vi "xml generate for SFP+_VNA_Full.vi"(0 "width1":dbl, 1 "width2":dbl, 2 "single spec":T1={"limit Spec"=array1616x8[12928 elements], "Diff Test Item Name"=["SDD21", "SDD11", "SCD22", "SCC11", "SCD21-SDD21", "NEXT", "ILD_15"], "Spec _Col"=[1, 2, 3, 4, 5, 6, 7]}, 3 "auto get refer point":bool, 4 "input_array_TDD11":string[](array[string]), 5 "input_array_TDD22":string[](array[string]), 6 "input_path_dataSource":path, 7 "input_test_results":bool[](array[boolean]), 8 "show_impspec":string[](array[string]), 10 "路径":path=path "D:/wmgxml.xml", 11 "input_array_time":string[](array[string]), 12 "input_str_label":string, 13 "input_array_impSpec":string[](array[string]), 14 "input_str_CustomerPN":string, 16 "FilePath":string, 17 "FileVer":string, 18 "terminal points":dbl[](array[numeric]), 19 "cable points":dbl[](array[numeric])) -> ()   [LabVIEW 2011]
uses:
  <vilib>/Utility/file.llb/Read From Spreadsheet File (DBL).vi
panel:
  out "terminal points 2":dbl[](array[numeric])
  out "TestResult":string
  out "TDD":string
  out "NEXT":string
  out "SCC11":string
  out "SCD21-SDD21":string
  out "ILD":string
  out "SDD11":string
  out "SDD21":string
  out "midVar_time":string[](array[string])
  in  "midVar_state":string
  in  "input_str_product":string
  out "midVar_Content":string
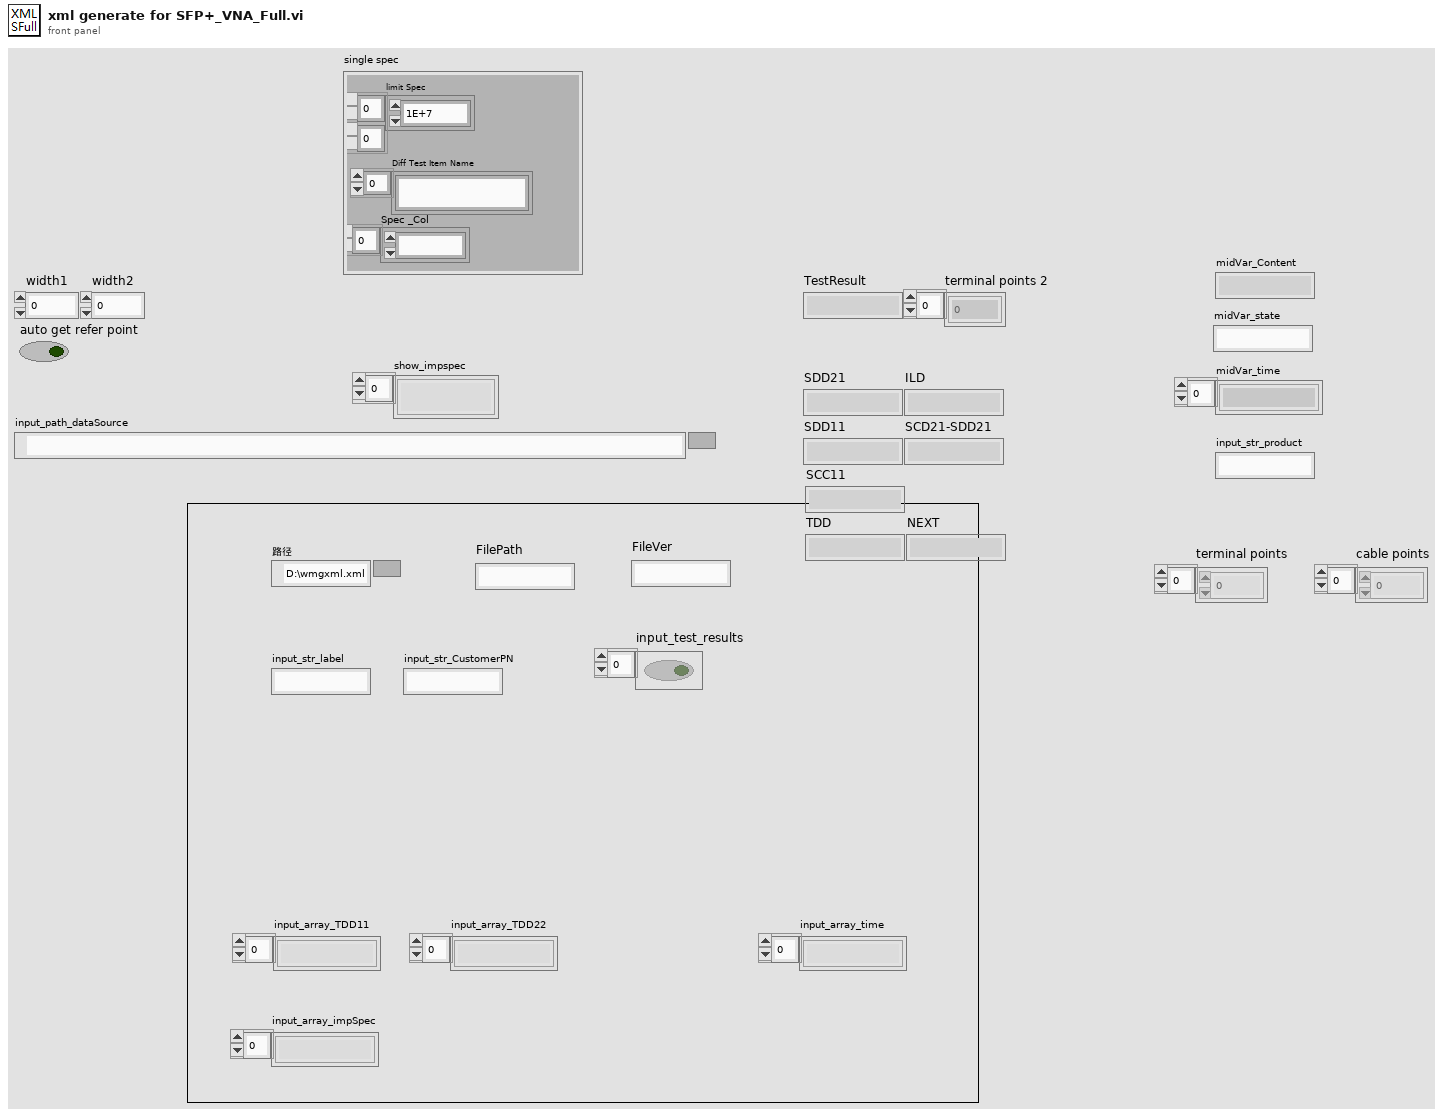
[diagram p1: front panel]
types:
  T1 = cluster{"limit Spec":dbl[][], "Diff Test Item Name":string[], "Spec _Col":i32[]}
  T2 = enum16{"open", "replace", "create", "open or create", "replace or create", "replace or create with confirmation"}
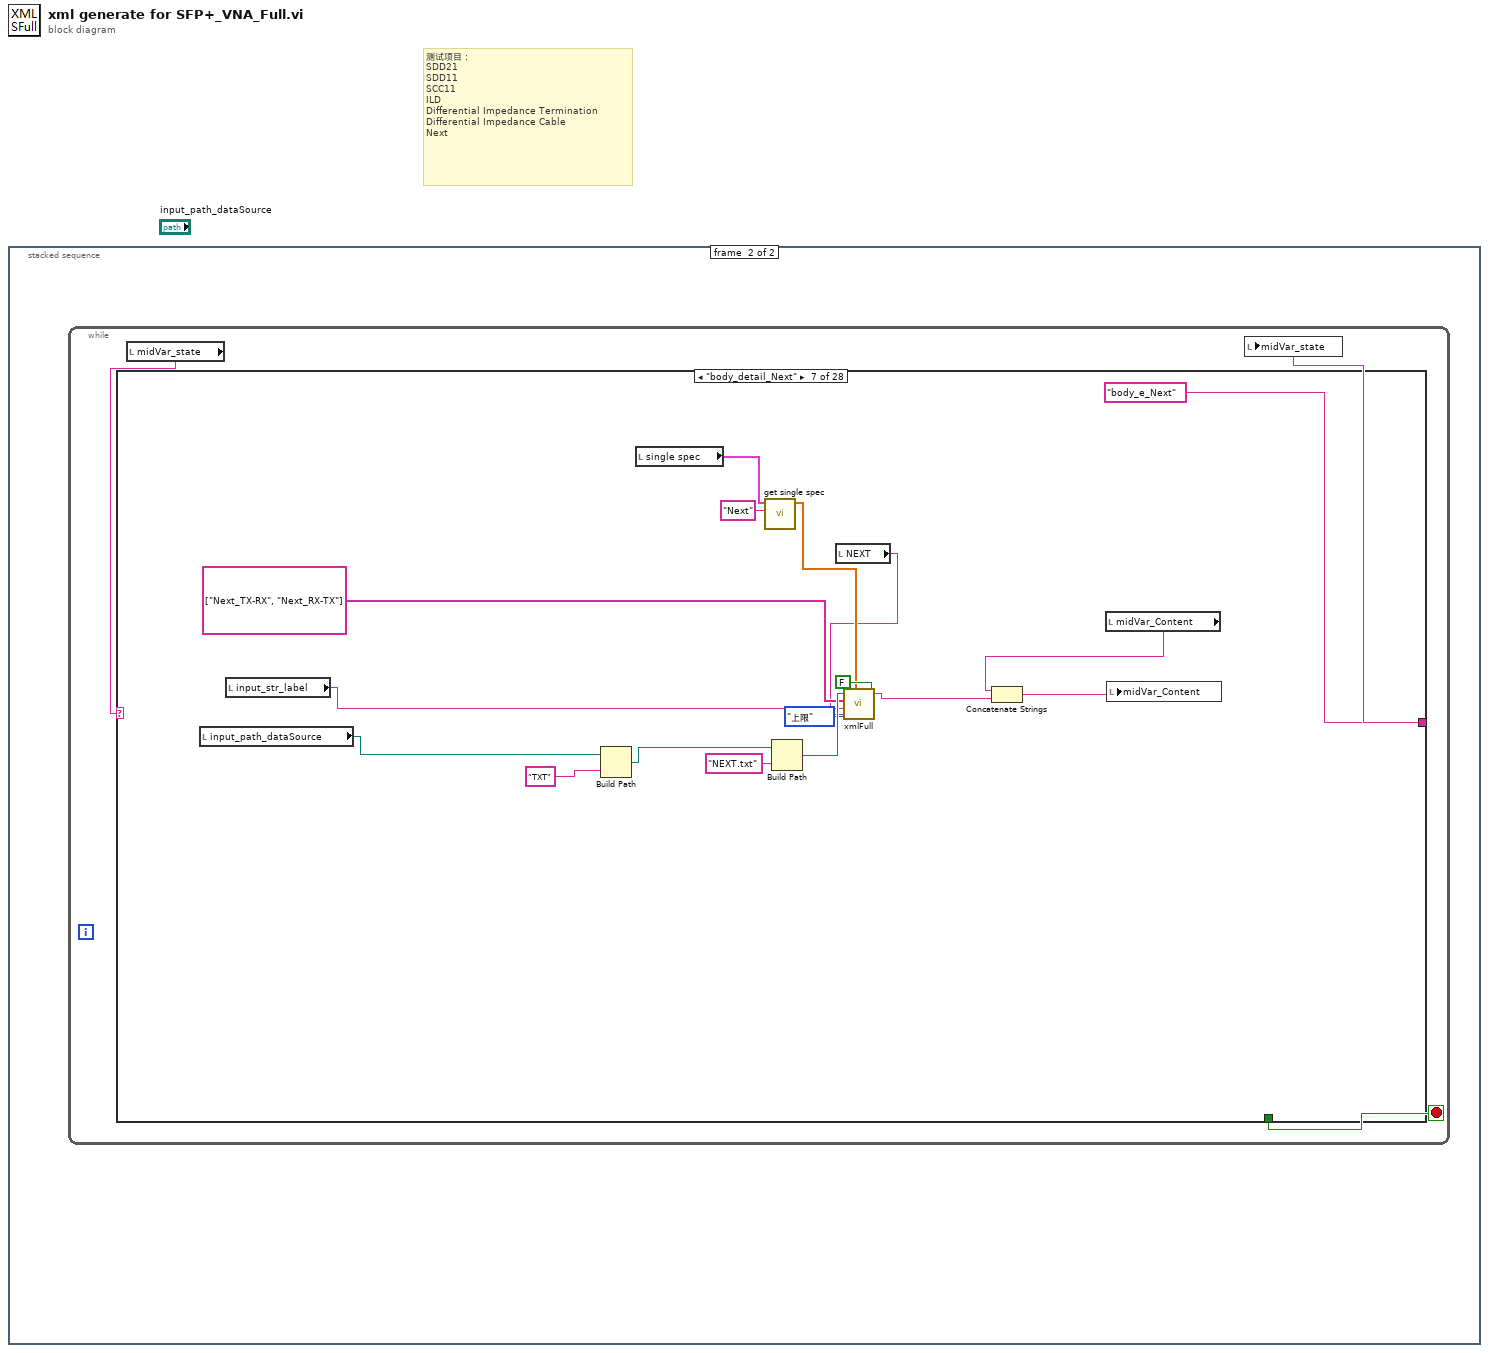
[diagram p0: block diagram]
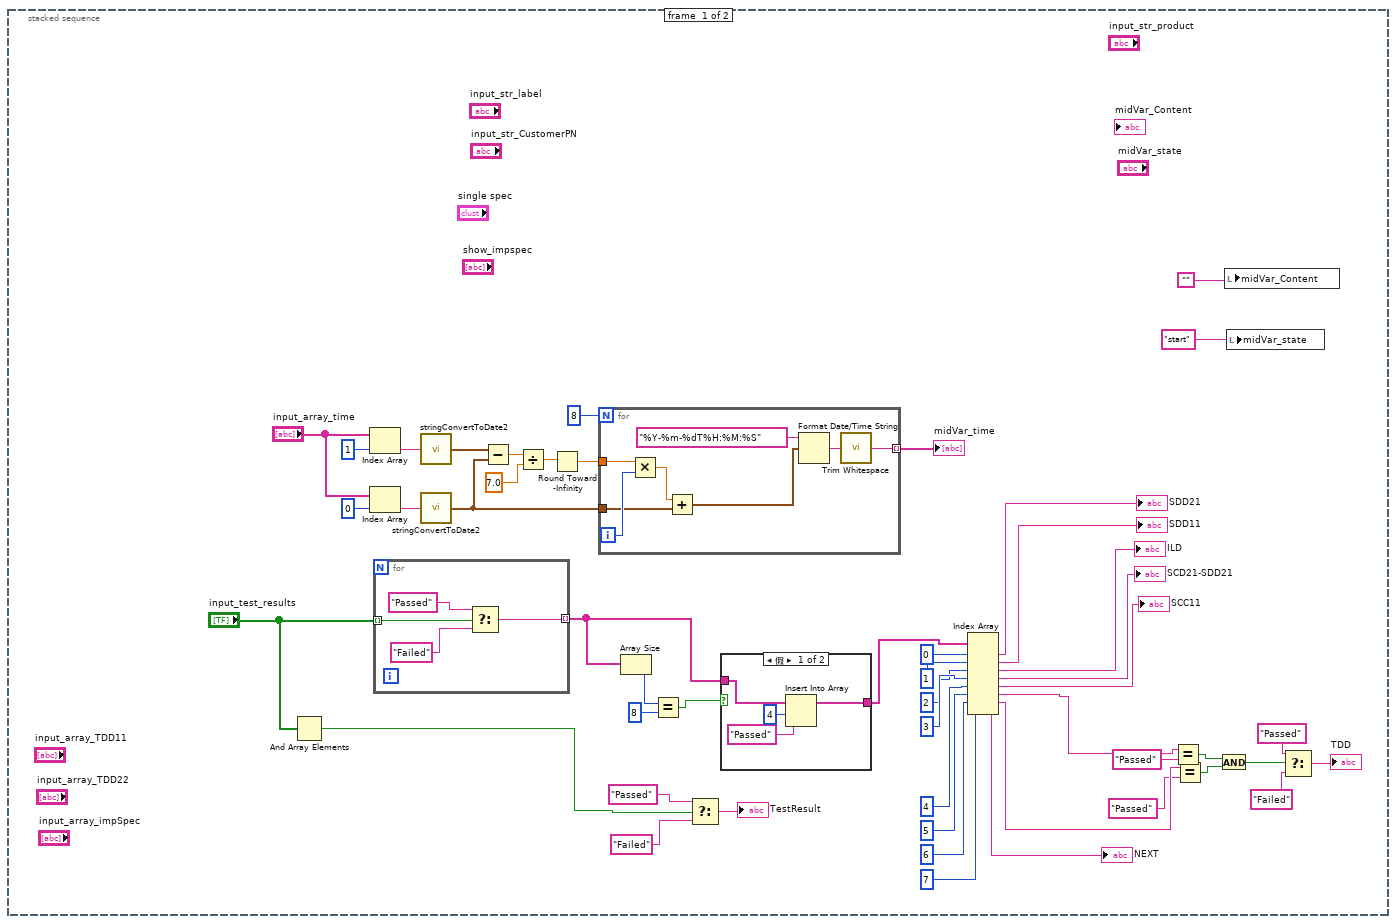
[diagram p2: hidden frame]
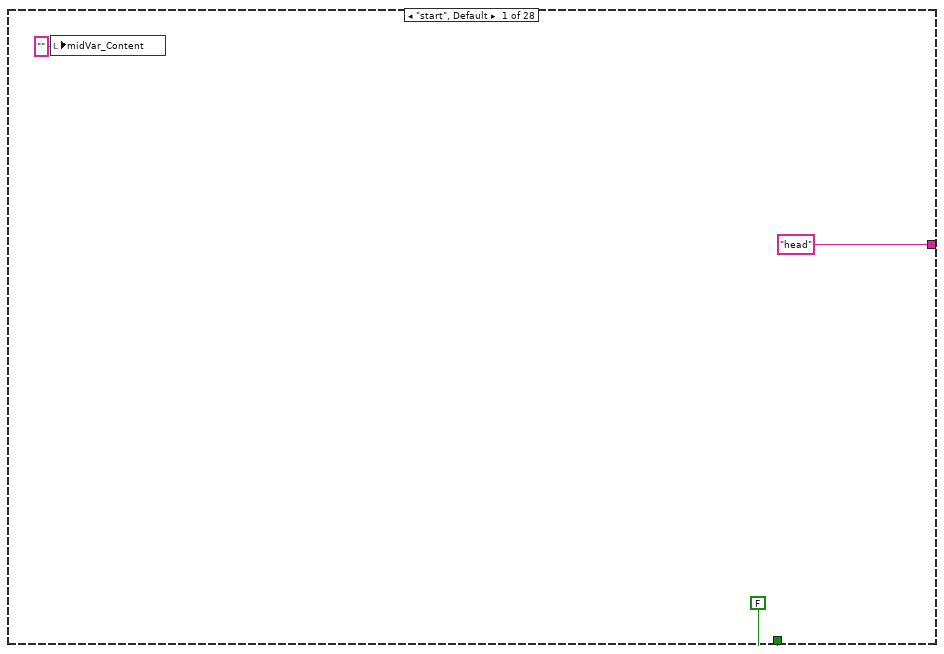
[diagram p4: hidden frame]
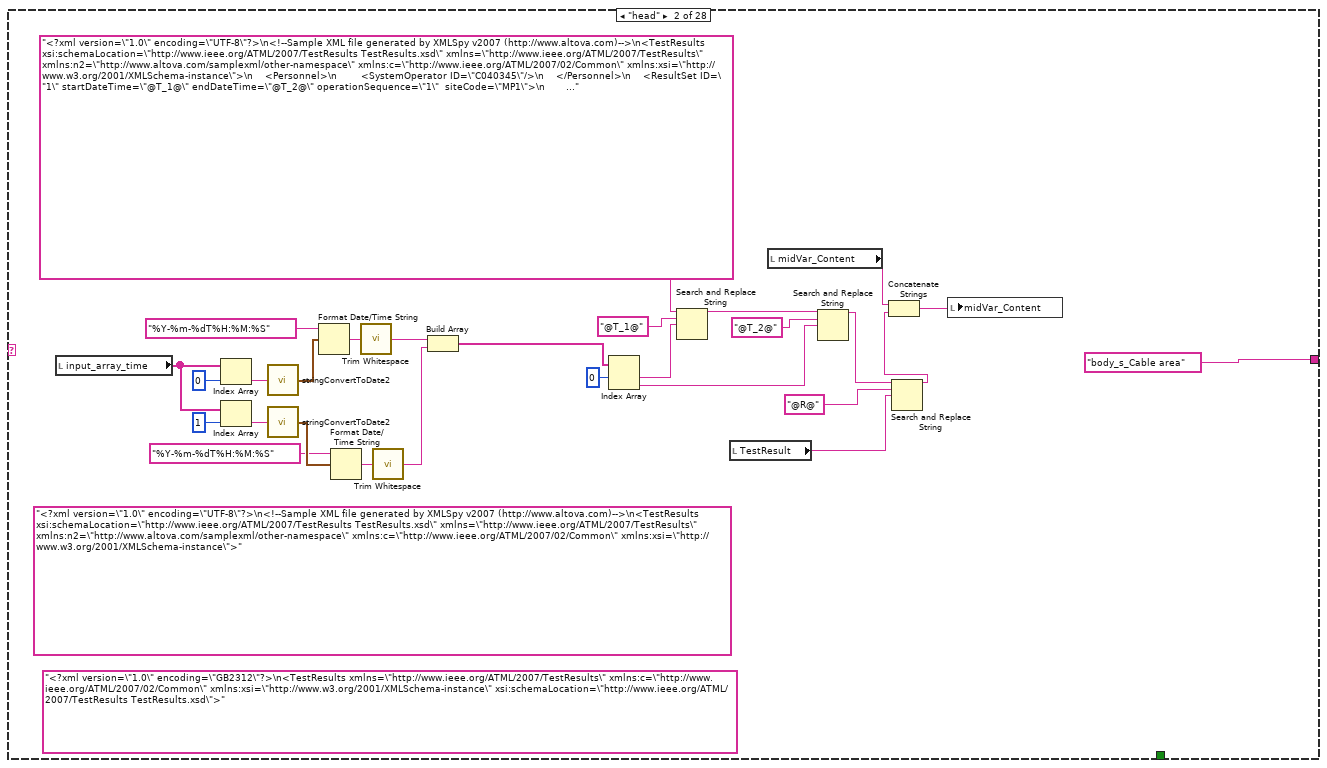
[diagram p5: hidden frame]
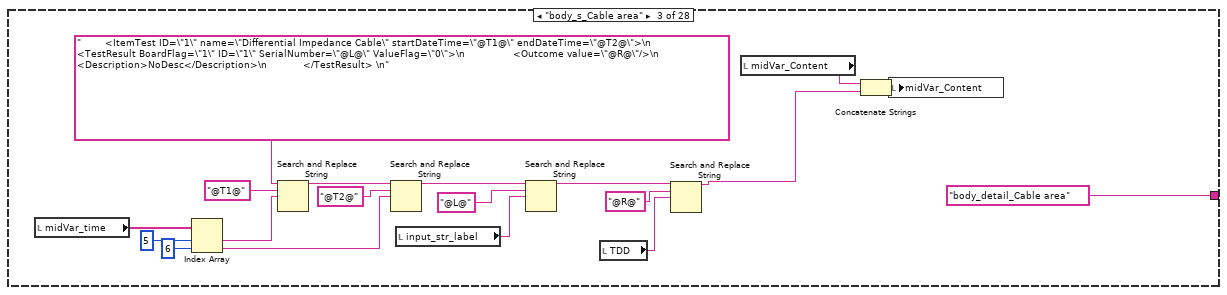
[diagram p6: hidden frame]
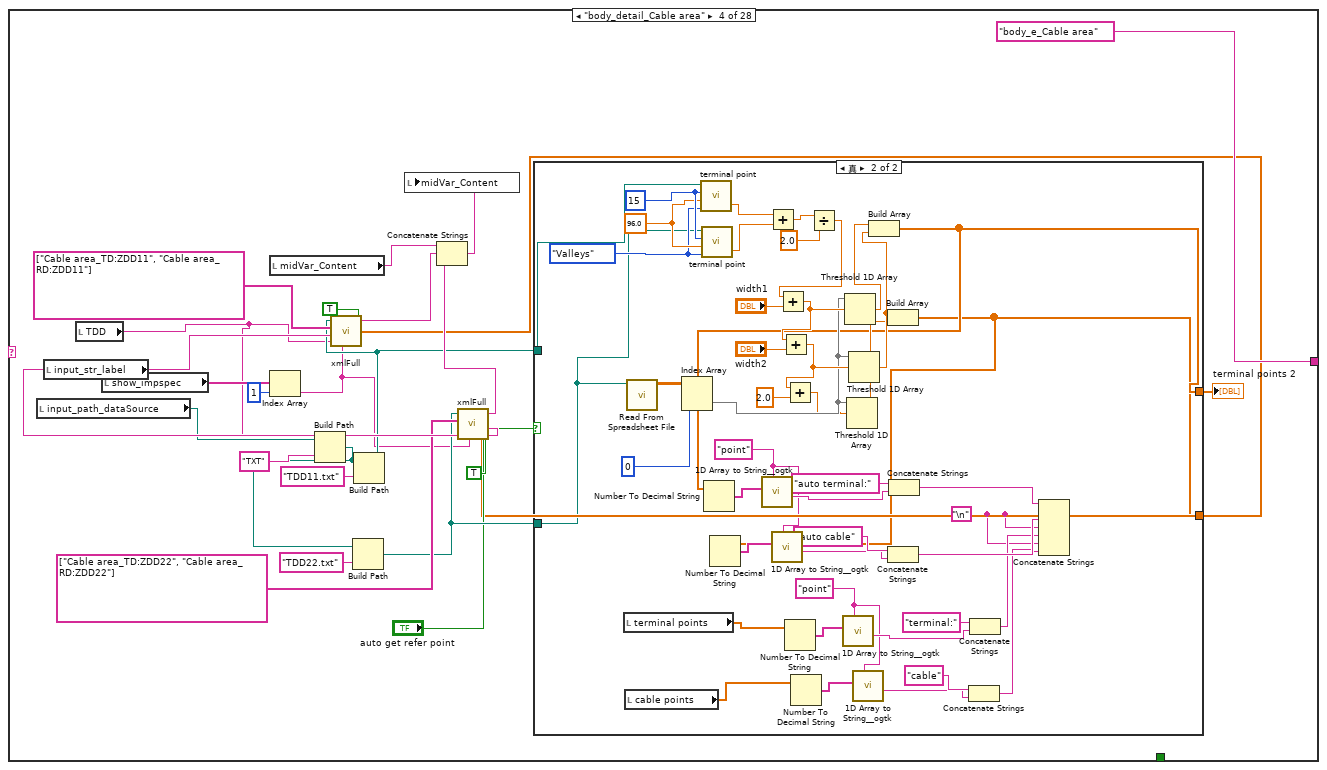
[diagram p7: hidden frame]
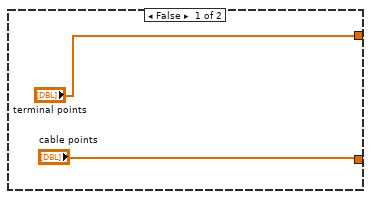
[diagram p8: hidden frame]
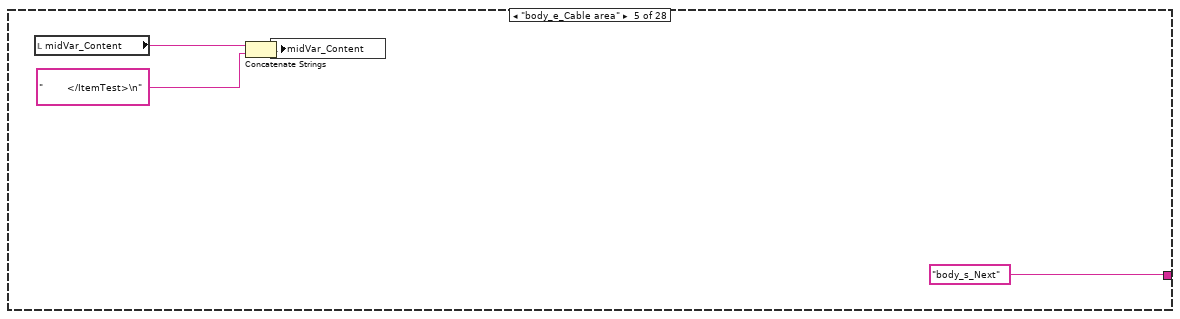
[diagram p9: hidden frame]
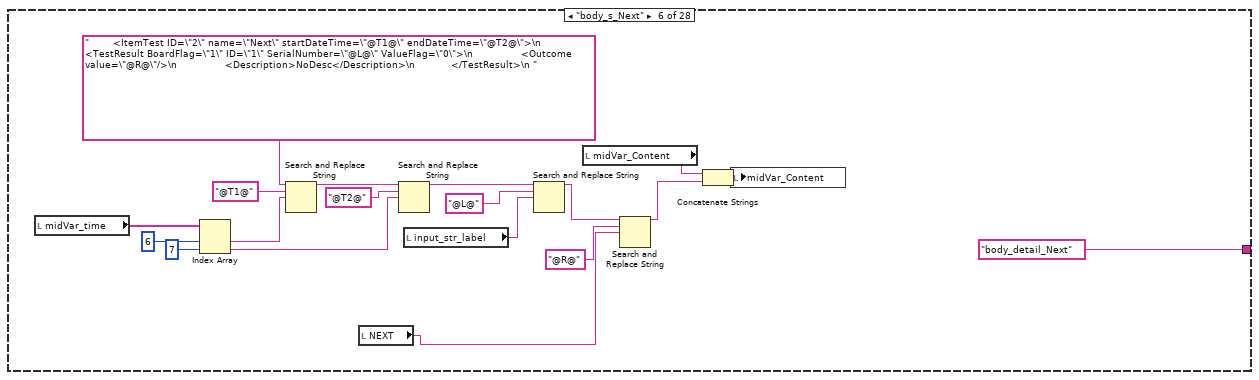
[diagram p10: hidden frame]
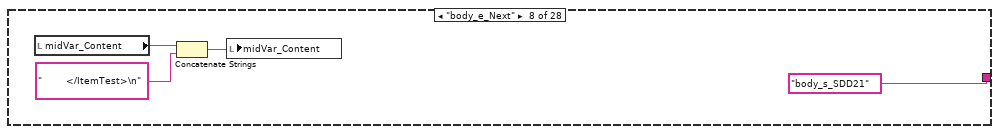
[diagram p11: hidden frame]
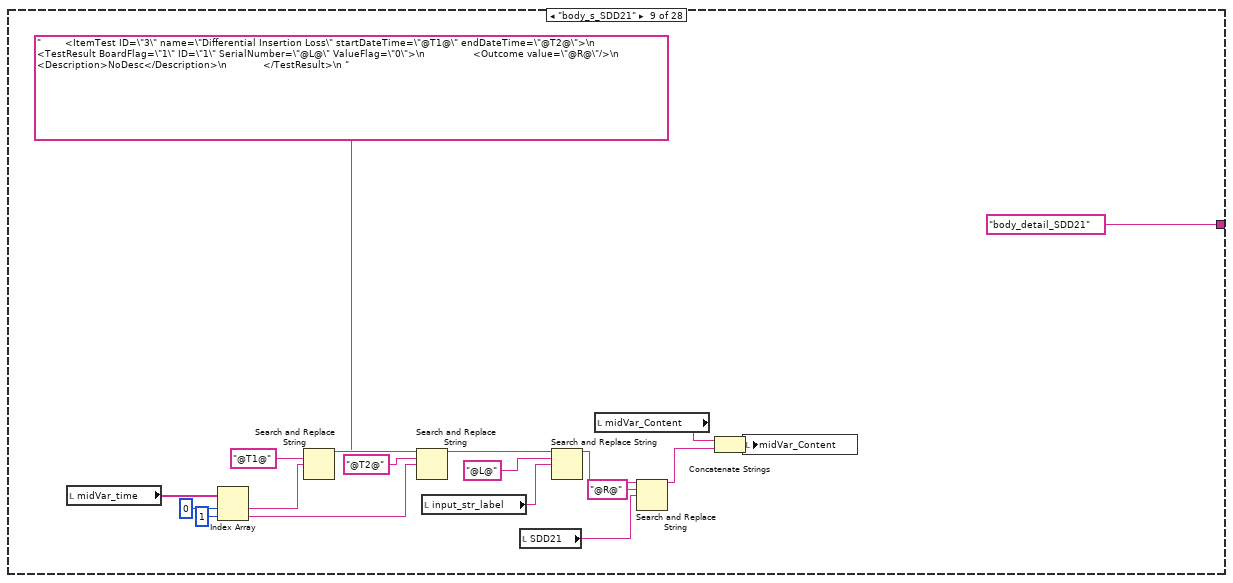
[diagram p12: hidden frame]
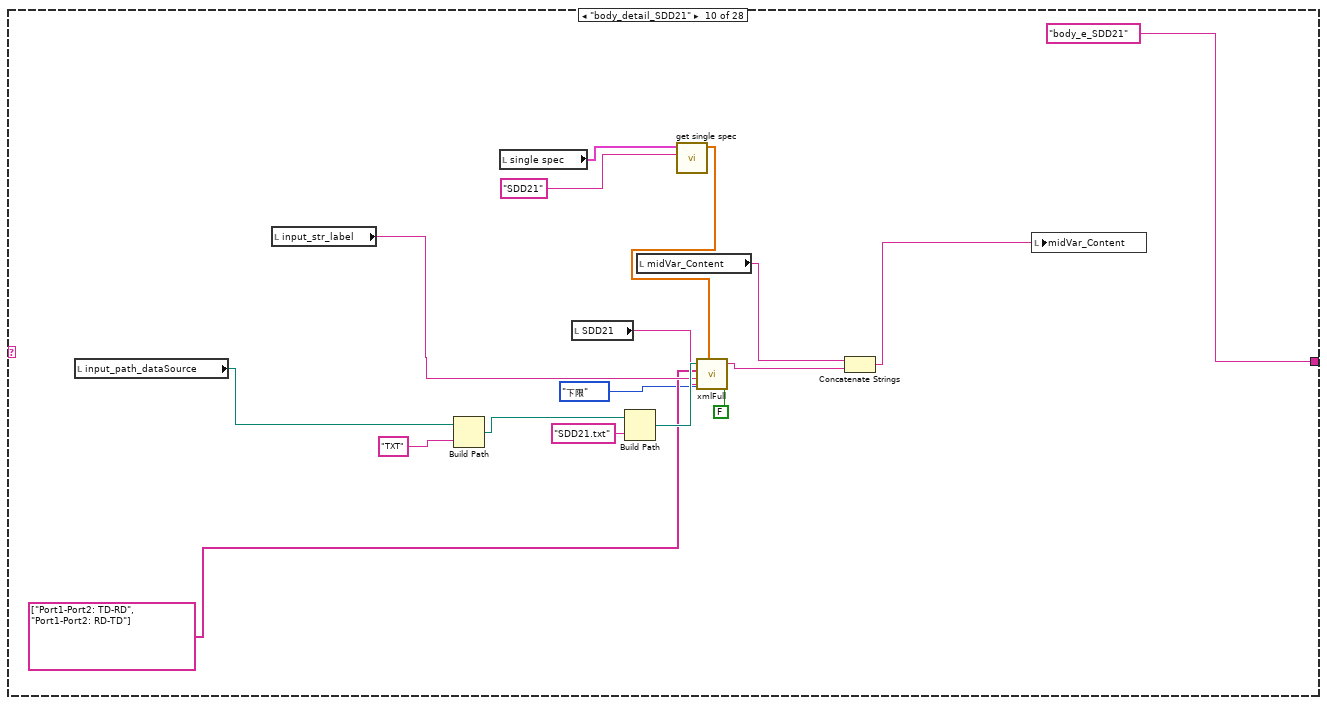
[diagram p13: hidden frame]
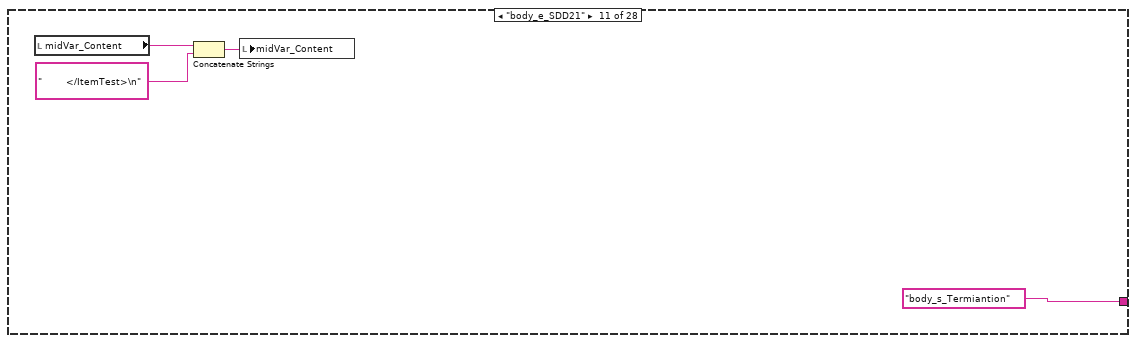
[diagram p14: hidden frame]
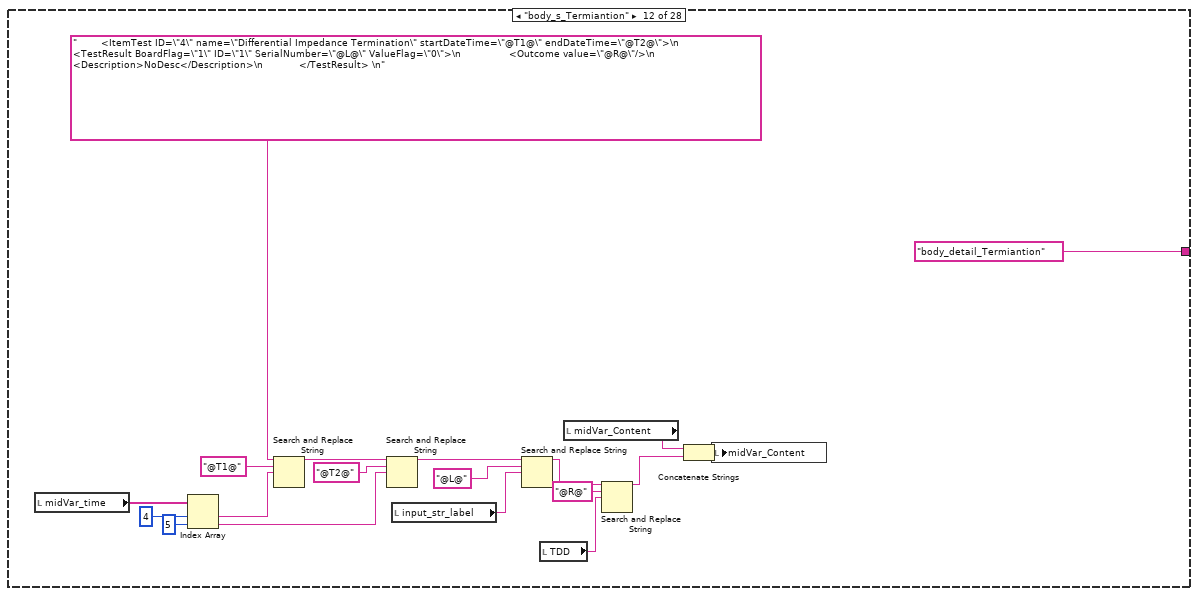
[diagram p15: hidden frame]
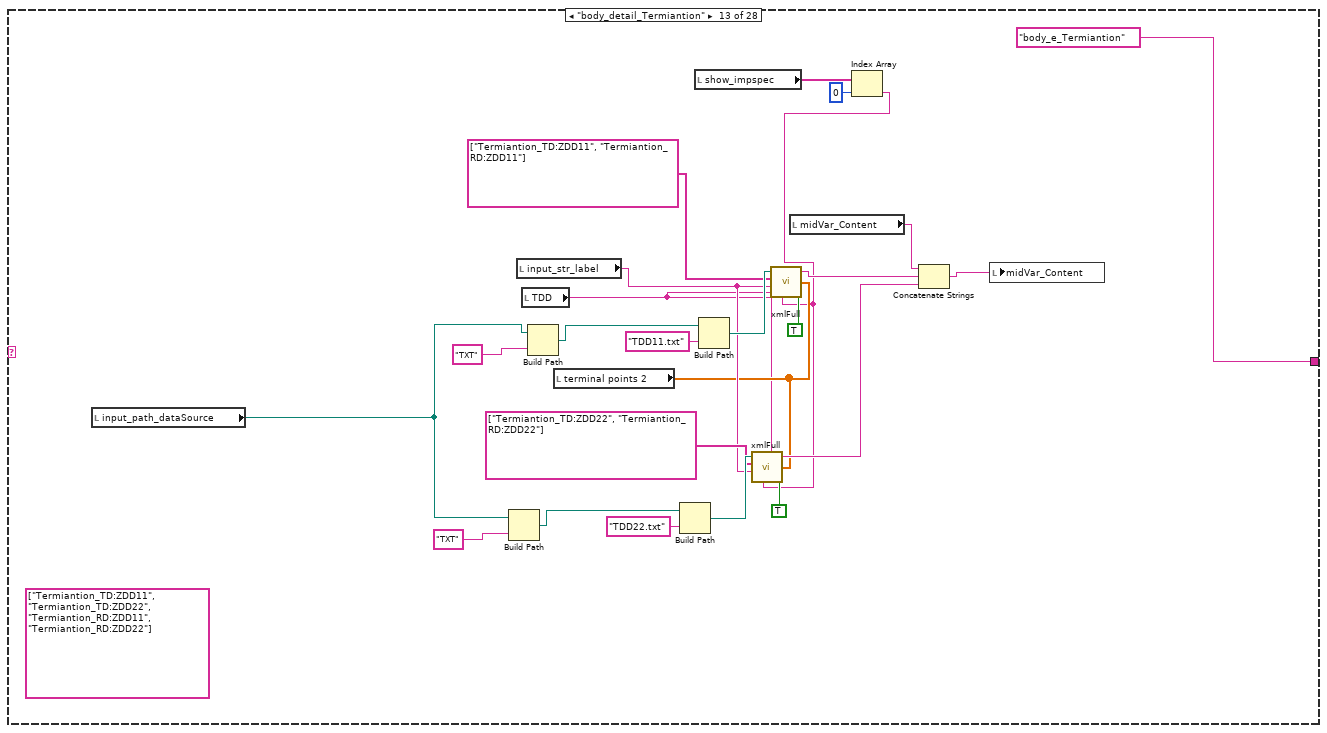
[diagram p16: hidden frame]
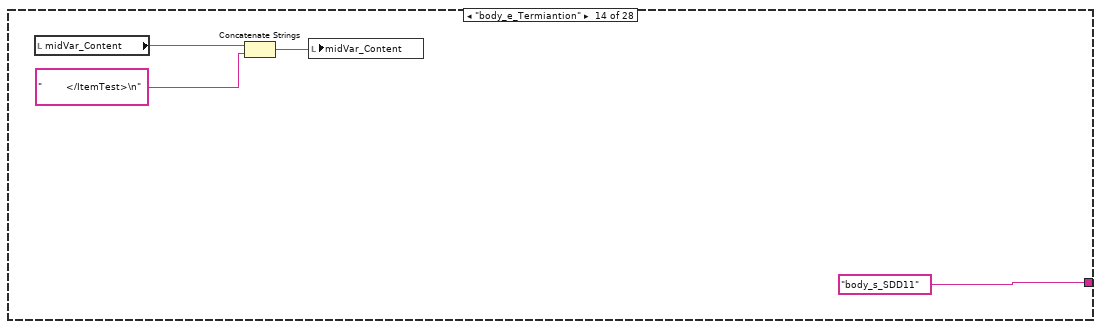
[diagram p17: hidden frame]
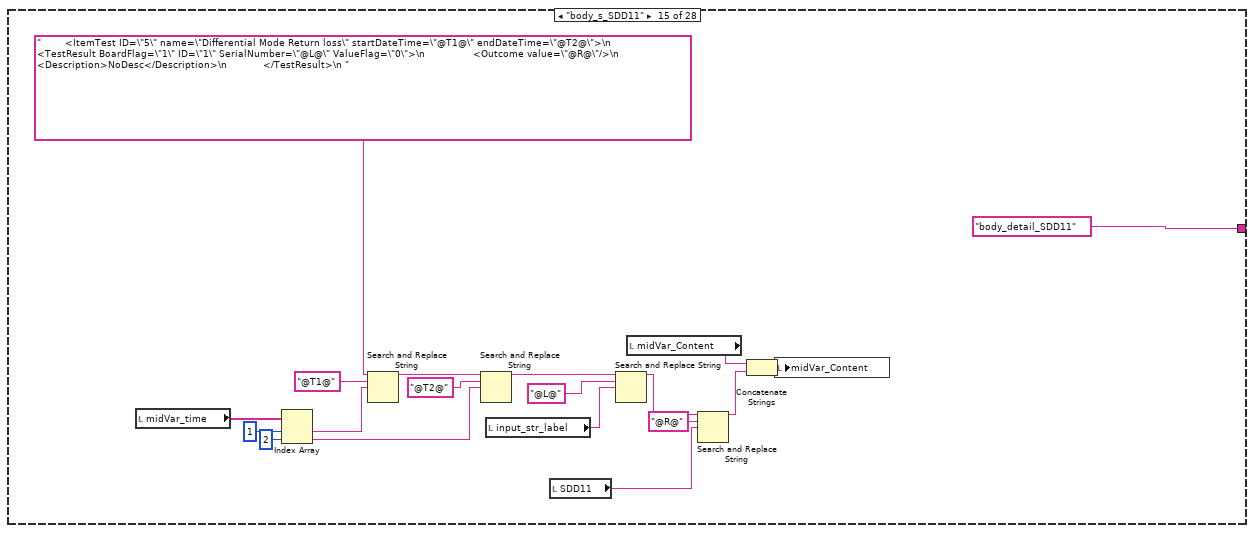
[diagram p18: hidden frame]
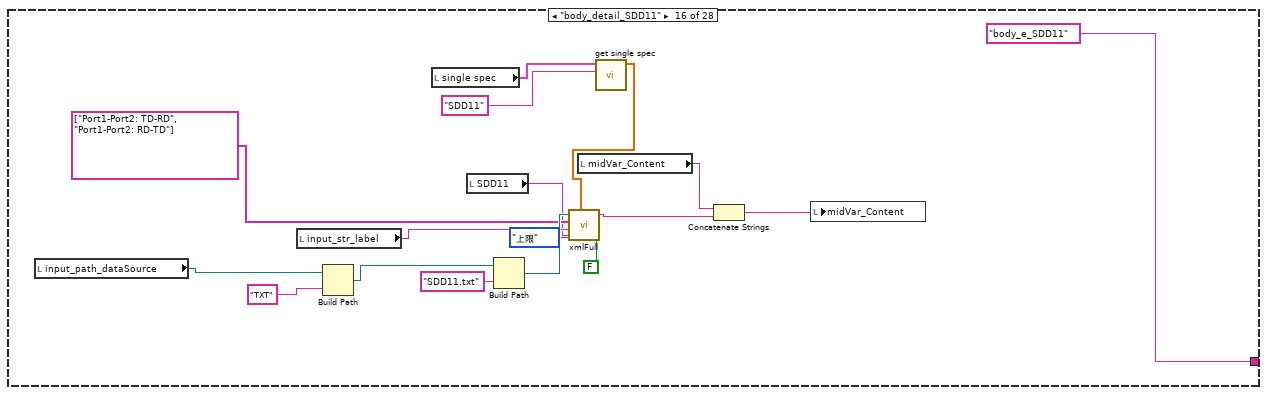
[diagram p19: hidden frame]
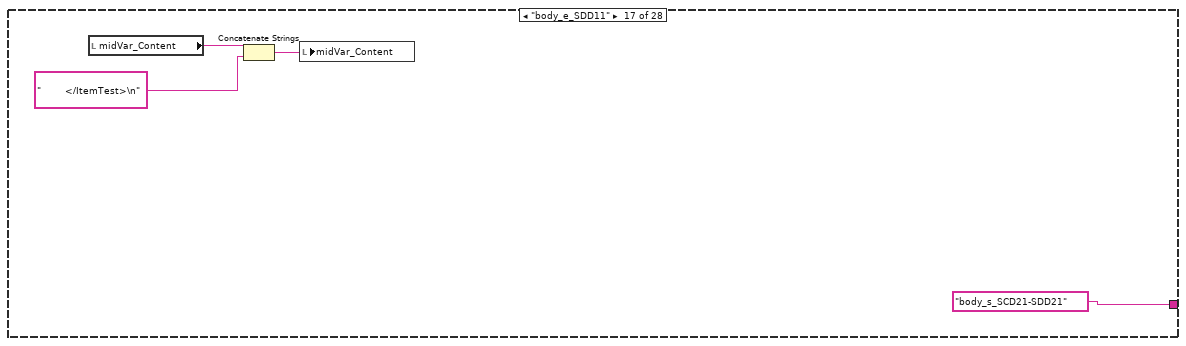
[diagram p20: hidden frame]
diagram:
  # "测试项目：\nSDD21\nSDD11\nSCC11\nILD\nDifferential Impedance Termination\nDifferential Impedance Cable\nNext"
  n1 = stacked-sequence {
    frame #0 {
      n2 = And Array Elements(Boolean array="input_test_results") -> (logical AND=w7:bool)
      n3 = Index Array(array="input_array_time", index=1 ("索引")) -> (element=w38:string)
      n4 = Index Array(array="input_array_time", index=0 ("索引")) -> (element=w39:string)
      n5 = for {
        tunnel: "input_test_results" -> [w58] mode=indexing
        tunnel: [w55] -> w2 mode=indexing
        n6 = Select(t="Passed", s=w58, f="Failed") -> (s? t:f=w55:string)
      }
      n7 = call "stringConvertToDate2.vi"("input_str_yymmdd"=w38) -> ("show_date"=w40:timestamp)
      n8 = call "stringConvertToDate2.vi"("input_str_yymmdd"=w39) -> ("show_date"=w46:timestamp)
      n9 = Subtract(x=w40, y=w46) -> (x-y=w41:dbl)
      n10 = Divide(x=w41, y=7.0) -> (x/y=w43:dbl)
      n11 = Round Toward -Infinity(1:w43) -> (0:w45:dbl)
      n12 = for {
        N: 8 -> [_]
        tunnel: w45 -> [w66]
        tunnel: w46 -> [w64]
        tunnel: [w59] -> w47 mode=indexing
        i -> [w65]
        n13 = Multiply(x=w66, y=w65) -> (x*y=w63:dbl)
        n14 = Add(x=w63, y=w64) -> (x+y=w60:timestamp)
        n15 = Format Date/Time String(time format string (%c)="%Y-%m-%dT%H:%M:%S" ("时间格式字符串(%c)"), seconds (now)=w60) -> (date/time string=w61:string)  [unwired: 1 in]
        n16 = call <vilib>:"Trim Whitespace.vi"("string"=w61) -> ("trimmed string"=w59:string)  [unwired: 1 in]
      }
      "midVar_time" <- w47
      n17 = Array Size(array=w2) -> (size(s)=w5:i32)
      n18 = Equal?(x=w5, y=8) -> (x = y?=w3:bool)
      n19 = Select(t="Passed", s=w7, f="Failed") -> (s? t:f=→"TestResult":string)
      n20 = case shown="假" w3 {
        tunnel: w2 -> [w53 w54]
        tunnel: [w50 w54] -> w1
        frame False {
          n21 = Insert Into Array(array=w53, index=4 ("索引"), new element="Passed" ("新元素/子数组")) -> (w50:string[])
        }
        frame True {
        }
      }
      n22 = Index Array(array=w1, index #1=0 ("索引"), index #2=1 ("索引"), index #3=2 ("索引"), index #4=3 ("索引"), index #5=4 ("索引"), index #6=5 ("索引"), index #7=6 ("索引"), index #8=7 ("索引")) -> (element #1=→"SDD21":string, element #2=→"SDD11":string, element #3=→"ILD":string, element #4=→"SCD21-SDD21":string, element #5=→"SCC11":string, element #6=w20:string, element #7=w18:string, element #8=→"NEXT":string)
      n23 = Equal?(x=w20, y="Passed") -> (x = y?=w16:bool)
      n24 = Equal?(x=w18, y="Passed") -> (x = y?=w15:bool)
      n25 = And(x=w16, y=w15) -> (x .and. y?=w14:bool)
      n26 = local write "midVar_Content"("") -> ()
      n27 = local write "midVar_state"("start" ("state")) -> ()
      n28 = Select(t="Passed", s=w14, f="Failed") -> (s? t:f=→"TDD":string)
    }
    frame #1 {
      n29 = while {
        stop <- w67 stop-if-true
        n30 = local read "midVar_state"() -> (w69:string)
        n31 = case shown="\"body_detail_Next\"" w69 {
          tunnel: ["head" ("state") "body_s_Cable area" ("state") "body_detail_Cable area" "body_e_Cable area" "body_s_Next" "body_detail_Next" "body_e_Next" "body_s_SDD21" "body_detail_SDD21" "body_e_SDD21" "body_s_Termiantion" "body_detail_Termiantion" "body_e_Termiantion" "body_s_SDD11" "body_detail_SDD11" "body_e_SDD11" "body_s_SCD21-SDD21" "body_detail_SCD21-SDD21" "body_e_SCD21-SDD21" "body_s_paddle card" "body_detail_paddle card" ("state") "body_e_paddle card" ("state") "body_s_ILD" ("state") "body_detail_ILD" "body_e_ILD" "tail" "end" ("state") "start" ("state")] -> w68
          tunnel: [FALSE _ _ _ _ _ _ _ _ _ _ _ _ _ _ _ _ _ _ _ _ _ _ _ _ _ _ TRUE] -> w67
          frame "start", Default {
            n32 = local write "midVar_Content"("" ("字符串")) -> ()
          }
          frame "head" {
            (unwired) "<?xml version=\"1.0\" encoding=\"GB2312\"?>\n<TestResults xmlns=\"http://www.ieee.org/ATML/2007/TestResults\" xmlns:c=\"http://www.ieee.org/ATML/2007/02/Common\" xmlns:xsi=\"http://www.w3.org/2001/XMLSchema-instance\" xsi:schemaLocation=\"http://www.ieee.org/ATML/2007/TestResults TestResults.xsd\">"
            (unwired) "<?xml version=\"1.0\" encoding=\"UTF-8\"?>\n<!--Sample XML file generated by XMLSpy v2007 (http://www.altova.com)-->\n<TestResults xsi:schemaLocation=\"http://www.ieee.org/ATML/2007/TestResults TestResults.xsd\" xmlns=\"http://www.ieee.org/ATML/2007/TestResults\" xmlns:n2=\"http://www.altova.com/samplexml/other-namespace\" xmlns:c=\"http://www.ieee.org/ATML/2007/02/Common\" xmlns:xsi=\"http://www.w3.org/2001/XMLSchema-instance\">"
            n33 = local read "input_array_time"() -> (w86:string[])
            n34 = Index Array(array=w86, index=0 ("索引")) -> (element=w85:string)
            n35 = Index Array(array=w86, index=1 ("索引")) -> (element=w84:string)
            n36 = call "stringConvertToDate2.vi"("input_str_yymmdd"=w85) -> ("show_date"=w82:timestamp)
            n37 = call "stringConvertToDate2.vi"("input_str_yymmdd"=w84) -> ("show_date"=w81:timestamp)
            n38 = Format Date/Time String(time format string (%c)="%Y-%m-%dT%H:%M:%S" ("时间格式字符串(%c)"), seconds (now)=w82) -> (date/time string=w89:string)  [unwired: 1 in]
            n39 = Format Date/Time String(time format string (%c)="%Y-%m-%dT%H:%M:%S" ("时间格式字符串(%c)"), seconds (now)=w81) -> (date/time string=w83:string)  [unwired: 1 in]
            n40 = call <vilib>:"Trim Whitespace.vi"("string"=w89) -> ("trimmed string"=w79:string)  [unwired: 1 in]
            n41 = call <vilib>:"Trim Whitespace.vi"("string"=w83) -> ("trimmed string"=w78:string)  [unwired: 1 in]
            n42 = Build Array(w79, w78) -> (w77:string[])
            n43 = Index Array(array=w77, index #1=0 ("索引")) -> (element #1=w98:string, element #2=w95:string)  [unwired: 1 in]
            n44 = Search and Replace String(input string="<?xml version=\"1.0\" encoding=\"UTF-8\"?>\n<!--Sample XML file generated by XMLSpy v2007 (http://www.altova.com)-->\n<TestResults xsi:schemaLocation=\"http://www.ieee.org/ATML/2007/TestResults TestResults.xsd\" xmlns=\"http://www.ieee.org/ATML/2007/TestResults\" xmlns:n2=\"http://www.altova.com/samplexml/other-namespace\" xmlns:c=\"http://www.ieee.org/ATML/2007/02/Common\" xmlns:xsi=\"http://www.w3.org/2001/XMLSchema-instance\">\n    <Personnel>\n        <SystemOperator ID=\"C040345\"/>\n    </Personnel>\n    <ResultSet ID=\"1\" startDateTime=\"@T_1@\" endDateTime=\"@T_2@\" operationSequence=\"1\"  siteCode=\"MP1\">\n        <Description>CMZ00A2R</Description>\n        <TestResult BoardFlag=\"1\" ID=\"1\">\n            <Outcome value=\"@R@\"/>\n        </TestResult>\n", search string="@T_1@" ("搜索字符串"), replace string=w98) -> (result string=w97:string)  [unwired: 5 in, 3 out]
            n45 = local read "TestResult"() -> (w73:string)
            n46 = local read "midVar_Content"() -> (w93:string)
            n47 = Search and Replace String(input string=w97, search string="@T_2@" ("搜索字符串"), replace string=w95) -> (result string=w76:string)  [unwired: 5 in, 3 out]
            n48 = Search and Replace String(input string=w76, search string="@R@" ("搜索字符串"), replace string=w73) -> (result string=w75:string)  [unwired: 5 in, 3 out]
            n49 = Concatenate Strings(w93, w75) -> (w92:string)
            n50 = local write "midVar_Content"(w92) -> ()
          }
          frame "body_s_Cable area" {
            n51 = local read "midVar_time"() -> (w106:string[])
            n52 = Index Array(array=w106, index #1=5 ("索引"), index #2=6 ("索引")) -> (element #1=w117:string, element #2=w114:string)
            n53 = Search and Replace String(input string="        <ItemTest ID=\"1\" name=\"Differential Impedance Cable\" startDateTime=\"@T1@\" endDateTime=\"@T2@\">\n            <TestResult BoardFlag=\"1\" ID=\"1\" SerialNumber=\"@L@\" ValueFlag=\"0\">\n                <Outcome value=\"@R@\"/>\n                <Description>NoDesc</Description>\n            </TestResult> \n", search string="@T1@" ("搜索字符串"), replace string=w117) -> (result string=w116:string)  [unwired: 5 in, 3 out]
            n54 = Search and Replace String(input string=w116, search string="@T2@" ("搜索字符串"), replace string=w114) -> (result string=w109:string)  [unwired: 5 in, 3 out]
            n55 = local read "input_str_label"() -> (w108:string)
            n56 = Search and Replace String(input string=w109, search string="@L@" ("搜索字符串"), replace string=w108) -> (result string=w104:string)  [unwired: 5 in, 3 out]
            n57 = local read "TDD"() -> (w101:string)
            n58 = Search and Replace String(input string=w104, search string="@R@" ("搜索字符串"), replace string=w101) -> (result string=w103:string)  [unwired: 5 in, 3 out]
            n59 = local read "midVar_Content"() -> (w113:string)
            n60 = Concatenate Strings(w113, w103) -> (w112:string)
            n61 = local write "midVar_Content"(w112) -> ()
          }
          frame "body_detail_Cable area" {
            n62 = local read "input_path_dataSource"() -> (w132:path)
            n63 = local read "input_str_label"() -> (w135:string)
            n64 = local read "TDD"() -> (w121:string)
            n65 = local read "show_impspec"() -> (w123:string[])
            n66 = local read "midVar_Content"() -> (w142:string)
            n67 = Index Array(array=w123, index=1 ("索引")) -> (element=w120:string)
            n68 = Build Path(base path=w132, name or relative path="TXT" ("名称或相对路径")) -> (appended path=w131:path)
            n69 = Build Path(base path=w131, name or relative path="TDD22.txt" ("名称或相对路径")) -> (appended path=w128:path)
            n70 = Build Path(base path=w131, name or relative path="TDD11.txt" ("名称或相对路径")) -> (appended path=w127:path)
            n71 = case shown="真" "auto get refer point" {
              tunnel: w128 -> [_ w178]
              tunnel: w127 -> [_ w190]
              tunnel: ["cable points" w151] -> w124
              tunnel: ["terminal points" w152] -> w125
              frame False {
              }
              frame True {
                w147 = "\n"
                w155 = "point" ("delimiter (Tab)")
                w164 = "point" ("delimiter (Tab)")
                w187 = enum32{"Peaks", "Valleys"}."Valleys" ("peaks/valleys")
                w188 = 96.0 ("threshold")
                w189 = 15 ("PD width")
                n72 = local read "terminal points"() -> (w160:dbl[])
                n73 = local read "cable points"() -> (w161:dbl[])
                n74 = call-poly <vilib>:"Read From Spreadsheet File.vi"("file path (dialog if empty)"=w178) -> ("all rows"=w177:dbl[][])  [unwired: 6 in, 4 out]
                n75 = Index Array(array=w177, index (col)=0 ("禁用的索引 (列)")) -> (element=w173:dbl[])  [unwired: 1 in]
                n76 = call "terminal point.vi"("peaks/valleys"=w187, "threshold"=w188, "PD width"=w189, "TDD filePath"=w190) -> ("time low"=w182:dbl)  [unwired: 1 out]
                n77 = call "terminal point.vi"("peaks/valleys"=w187, "threshold"=w188, "PD width"=w189, "TDD filePath"=w178) -> ("time low"=w181:dbl)  [unwired: 1 out]
                n78 = Add(x=w182, y=w181) -> (x+y=w186:dbl)
                n79 = Number To Decimal String(number=w160) -> (decimal integer string=w162:string[])  [unwired: 1 in]
                n80 = Number To Decimal String(number=w161) -> (decimal integer string=w163:string[])  [unwired: 1 in]
                n81 = Divide(x=w186, y=2.0) -> (x/y=w179:dbl)
                n82 = Add(x=w179, y="width1") -> (x+y=w175:dbl)
                n83 = Add(x=w175, y="width2") -> (x+y=w174:dbl)
                n84 = Add(x=w174, y=2.0) -> (x+y=w172:dbl)
                n85 = call <userlib>:"1D Array to String__ogtk.vi"("delimiter (Tab)"=w164, "Array of Strings"=w162) -> ("delimited string"=w166:string)  [unwired: 9 in]
                n86 = Threshold 1D Array(2:w175, 3:w173) -> (0:w171:dbl)  [unwired: 1 in]
                n87 = Threshold 1D Array(2:w172, 3:w173) -> (0:w169:dbl)  [unwired: 1 in]
                n88 = Threshold 1D Array(2:w174, 3:w173) -> (0:w170:dbl)  [unwired: 1 in]
                n89 = call <userlib>:"1D Array to String__ogtk.vi"("delimiter (Tab)"=w164, "Array of Strings"=w163) -> ("delimited string"=w167:string)  [unwired: 9 in]
                n90 = Build Array(w171, w170) -> (w152:dbl[])
                n91 = Number To Decimal String(number=w152) -> (decimal integer string=w153:string[])  [unwired: 1 in]
                n92 = call <userlib>:"1D Array to String__ogtk.vi"("delimiter (Tab)"=w155, "Array of Strings"=w153) -> ("delimited string"=w157:string)  [unwired: 9 in]
                n93 = Build Array(w170, w169) -> (w151:dbl[])
                n94 = Number To Decimal String(number=w151) -> (decimal integer string=w154:string[])  [unwired: 1 in]
                n95 = call <userlib>:"1D Array to String__ogtk.vi"("delimiter (Tab)"=w155, "Array of Strings"=w154) -> ("delimited string"=w158:string)  [unwired: 9 in]
                n96 = Concatenate Strings("auto cable" ("字符串"), w158) -> (w149:string)
                n97 = Concatenate Strings("auto terminal:" ("字符串"), w157) -> (w150:string)
                n98 = Concatenate Strings("cable" ("字符串"), w167) -> (w146:string)
                n99 = Concatenate Strings("terminal:" ("字符串"), w166) -> (w148:string)
                n100 = Concatenate Strings(w150, w147, w149, w147, w148, w147, w146) -> ()  [unwired: 1 out]
              }
            }
            "terminal points 2" <- w125
            n101 = call "xmlFull.vi"("TDD?"=TRUE, "second result"=w121, "Points"=w124, "file path (dialog if empty)"=w127, "TDD spec"=w120, "SN"=w135, "数组"=string[] ["Cable area_TD:ZDD11", "Cable area_RD:ZDD11"]) -> ("OutPutXml"=w140:string)  [unwired: 3 in]
            n102 = call "xmlFull.vi"("TDD?"=TRUE, "second result"=w121, "Points"=w124, "file path (dialog if empty)"=w128, "TDD spec"=w120, "SN"=w135, "数组"=string[] ["Cable area_TD:ZDD22", "Cable area_RD:ZDD22"]) -> ("OutPutXml"=w133:string)  [unwired: 3 in]
            n103 = Concatenate Strings(w142, w140, w133) -> (w141:string)
            n104 = local write "midVar_Content"(w141) -> ()
          }
          frame "body_e_Cable area" {
            n105 = local read "midVar_Content"() -> (w194:string)
            n106 = Concatenate Strings(w194, "        </ItemTest>\n") -> (w193:string)
            n107 = local write "midVar_Content"(w193) -> ()
          }
          frame "body_s_Next" {
            n108 = local read "midVar_time"() -> (w200:string[])
            n109 = Index Array(array=w200, index #1=6 ("索引"), index #2=7 ("索引")) -> (element #1=w211:string, element #2=w208:string)
            n110 = Search and Replace String(input string="        <ItemTest ID=\"2\" name=\"Next\" startDateTime=\"@T1@\" endDateTime=\"@T2@\">\n            <TestResult BoardFlag=\"1\" ID=\"1\" SerialNumber=\"@L@\" ValueFlag=\"0\">\n                <Outcome value=\"@R@\"/>\n                <Description>NoDesc</Description>\n            </TestResult>\n ", search string="@T1@" ("搜索字符串"), replace string=w211) -> (result string=w210:string)  [unwired: 5 in, 3 out]
            n111 = local read "NEXT"() -> (w198:string)
            n112 = Search and Replace String(input string=w210, search string="@T2@" ("搜索字符串"), replace string=w208) -> (result string=w203:string)  [unwired: 5 in, 3 out]
            n113 = local read "input_str_label"() -> (w202:string)
            n114 = Search and Replace String(input string=w203, search string="@L@" ("搜索字符串"), replace string=w202) -> (result string=w196:string)  [unwired: 5 in, 3 out]
            n115 = local read "midVar_Content"() -> (w207:string)
            n116 = Search and Replace String(input string=w196, search string="@R@" ("搜索字符串"), replace string=w198) -> (result string=w195:string)  [unwired: 5 in, 3 out]
            n117 = Concatenate Strings(w207, w195) -> (w206:string)
            n118 = local write "midVar_Content"(w206) -> ()
          }
          frame "body_detail_Next" {
            n119 = local read "input_path_dataSource"() -> (w226:path)
            n120 = local read "input_str_label"() -> (w224:string)
            n121 = Build Path(base path=w226, name or relative path="TXT" ("名称或相对路径")) -> (appended path=w228:path)
            n122 = local read "single spec"() -> (w217:T1)
            n123 = call "get single spec.vi"("single item name"="Next", "single spec"=w217) -> ("single spec"=w216:dbl[])  [unwired: 9 in]
            n124 = Build Path(base path=w228, name or relative path="NEXT.txt" ("名称或相对路径")) -> (appended path=w225:path)
            n125 = local read "NEXT"() -> (w215:string)
            n126 = call "xmlFull.vi"("TDD?"=FALSE, "second result"=w215, "file path (dialog if empty)"=w225, "limit type"=enum16{"上限", "下限"}."上限", "SN"=w224, "single spec"=w216, "数组"=string[] ["Next_TX-RX", "Next_RX-TX"]) -> ("OutPutXml"=w222:string)  [unwired: 3 in]
            n127 = local read "midVar_Content"() -> (w221:string)
            n128 = Concatenate Strings(w221, w222) -> (w220:string)
            n129 = local write "midVar_Content"(w220) -> ()
          }
          frame "body_e_Next" {
            n130 = local read "midVar_Content"() -> (w234:string)
            n131 = Concatenate Strings(w234, "        </ItemTest>\n") -> (w233:string)
            n132 = local write "midVar_Content"(w233) -> ()
          }
          frame "body_s_SDD21" {
            n133 = local read "midVar_time"() -> (w240:string[])
            n134 = Index Array(array=w240, index #1=0 ("索引"), index #2=1 ("索引")) -> (element #1=w251:string, element #2=w248:string)
            n135 = Search and Replace String(input string="        <ItemTest ID=\"3\" name=\"Differential Insertion Loss\" startDateTime=\"@T1@\" endDateTime=\"@T2@\">\n            <TestResult BoardFlag=\"1\" ID=\"1\" SerialNumber=\"@L@\" ValueFlag=\"0\">\n                <Outcome value=\"@R@\"/>\n                <Description>NoDesc</Description>\n            </TestResult>\n ", search string="@T1@" ("搜索字符串"), replace string=w251) -> (result string=w250:string)  [unwired: 5 in, 3 out]
            n136 = Search and Replace String(input string=w250, search string="@T2@" ("搜索字符串"), replace string=w248) -> (result string=w243:string)  [unwired: 5 in, 3 out]
            n137 = local read "input_str_label"() -> (w242:string)
            n138 = local read "SDD21"() -> (w235:string)
            n139 = Search and Replace String(input string=w243, search string="@L@" ("搜索字符串"), replace string=w242) -> (result string=w238:string)  [unwired: 5 in, 3 out]
            n140 = local read "midVar_Content"() -> (w247:string)
            n141 = Search and Replace String(input string=w238, search string="@R@" ("搜索字符串"), replace string=w235) -> (result string=w237:string)  [unwired: 5 in, 3 out]
            n142 = Concatenate Strings(w247, w237) -> (w246:string)
            n143 = local write "midVar_Content"(w246) -> ()
          }
          frame "body_detail_SDD21" {
            n144 = local read "input_path_dataSource"() -> (w264:path)
            n145 = local read "input_str_label"() -> (w263:string)
            n146 = Build Path(base path=w264, name or relative path="TXT" ("名称或相对路径")) -> (appended path=w268:path)
            n147 = local read "single spec"() -> (w257:T1)
            n148 = local read "SDD21"() -> (w258:string)
            n149 = Build Path(base path=w268, name or relative path="SDD21.txt" ("名称或相对路径")) -> (appended path=w266:path)
            n150 = local read "midVar_Content"() -> (w261:string)
            n151 = call "get single spec.vi"("single item name"="SDD21", "single spec"=w257) -> ("single spec"=w255:dbl[])  [unwired: 9 in]
            n152 = call "xmlFull.vi"("TDD?"=FALSE, "second result"=w258, "file path (dialog if empty)"=w266, "limit type"=enum16{"上限", "下限"}."下限", "SN"=w263, "single spec"=w255, "数组"=string[] ["Port1-Port2: TD-RD", "Port1-Port2: RD-TD"]) -> ("OutPutXml"=w265:string)  [unwired: 3 in]
            n153 = Concatenate Strings(w261, w265) -> (w262:string)
            n154 = local write "midVar_Content"(w262) -> ()
          }
          frame "body_e_SDD21" {
            n155 = local read "midVar_Content"() -> (w274:string)
            n156 = Concatenate Strings(w274, "        </ItemTest>\n") -> (w273:string)
            n157 = local write "midVar_Content"(w273) -> ()
          }
          frame "body_s_Termiantion" {
            n158 = local read "midVar_time"() -> (w280:string[])
            n159 = Index Array(array=w280, index #1=4 ("索引"), index #2=5 ("索引")) -> (element #1=w291:string, element #2=w288:string)
            n160 = Search and Replace String(input string="        <ItemTest ID=\"4\" name=\"Differential Impedance Termination\" startDateTime=\"@T1@\" endDateTime=\"@T2@\">\n            <TestResult BoardFlag=\"1\" ID=\"1\" SerialNumber=\"@L@\" ValueFlag=\"0\">\n                <Outcome value=\"@R@\"/>\n                <Description>NoDesc</Description>\n            </TestResult> \n", search string="@T1@" ("搜索字符串"), replace string=w291) -> (result string=w290:string)  [unwired: 5 in, 3 out]
            n161 = Search and Replace String(input string=w290, search string="@T2@" ("搜索字符串"), replace string=w288) -> (result string=w283:string)  [unwired: 5 in, 3 out]
            n162 = local read "input_str_label"() -> (w282:string)
            n163 = Search and Replace String(input string=w283, search string="@L@" ("搜索字符串"), replace string=w282) -> (result string=w278:string)  [unwired: 5 in, 3 out]
            n164 = local read "TDD"() -> (w275:string)
            n165 = local read "midVar_Content"() -> (w287:string)
            n166 = Search and Replace String(input string=w278, search string="@R@" ("搜索字符串"), replace string=w275) -> (result string=w277:string)  [unwired: 5 in, 3 out]
            n167 = Concatenate Strings(w287, w277) -> (w286:string)
            n168 = local write "midVar_Content"(w286) -> ()
          }
          frame "body_detail_Termiantion" {
            (unwired) string[] ["Termiantion_TD:ZDD11", "Termiantion_TD:ZDD22", "Termiantion_RD:ZDD11", "Termiantion_RD:ZDD22"]
            n169 = local read "input_path_dataSource"() -> (w304:path)
            n170 = Build Path(base path=w304, name or relative path="TXT" ("名称或相对路径")) -> (appended path=w311:path)
            n171 = local read "input_str_label"() -> (w301:string)
            n172 = local read "TDD"() -> (w297:string)
            n173 = Build Path(base path=w304, name or relative path="TXT" ("名称或相对路径")) -> (appended path=w315:path)
            n174 = local read "terminal points 2"() -> (w298:dbl[])
            n175 = Build Path(base path=w311, name or relative path="TDD22.txt" ("名称或相对路径")) -> (appended path=w309:path)
            n176 = local read "show_impspec"() -> (w296:string[])
            n177 = Build Path(base path=w315, name or relative path="TDD11.txt" ("名称或相对路径")) -> (appended path=w313:path)
            n178 = local read "midVar_Content"() -> (w299:string)
            n179 = Index Array(array=w296, index=0 ("索引")) -> (element=w294:string)
            n180 = call "xmlFull.vi"("TDD?"=TRUE, "second result"=w297, "Points"=w298, "file path (dialog if empty)"=w309, "TDD spec"=w294, "SN"=w301, "数组"=string[] ["Termiantion_TD:ZDD22", "Termiantion_RD:ZDD22"]) -> ("OutPutXml"=w307:string)  [unwired: 3 in]
            n181 = call "xmlFull.vi"("TDD?"=TRUE, "second result"=w297, "Points"=w298, "file path (dialog if empty)"=w313, "TDD spec"=w294, "SN"=w301, "数组"=string[] ["Termiantion_TD:ZDD11", "Termiantion_RD:ZDD11"]) -> ("OutPutXml"=w308:string)  [unwired: 3 in]
            n182 = Concatenate Strings(w299, w308, w307) -> (w300:string)
            n183 = local write "midVar_Content"(w300) -> ()
          }
          frame "body_e_Termiantion" {
            n184 = local read "midVar_Content"() -> (w321:string)
            n185 = Concatenate Strings(w321, "        </ItemTest>\n") -> (w320:string)
            n186 = local write "midVar_Content"(w320) -> ()
          }
          frame "body_s_SDD11" {
            n187 = local read "midVar_time"() -> (w327:string[])
            n188 = Index Array(array=w327, index #1=1 ("索引"), index #2=2 ("索引")) -> (element #1=w338:string, element #2=w335:string)
            n189 = Search and Replace String(input string="        <ItemTest ID=\"5\" name=\"Differential Mode Return loss\" startDateTime=\"@T1@\" endDateTime=\"@T2@\">\n            <TestResult BoardFlag=\"1\" ID=\"1\" SerialNumber=\"@L@\" ValueFlag=\"0\">\n                <Outcome value=\"@R@\"/>\n                <Description>NoDesc</Description>\n            </TestResult>\n ", search string="@T1@" ("搜索字符串"), replace string=w338) -> (result string=w337:string)  [unwired: 5 in, 3 out]
            n190 = Search and Replace String(input string=w337, search string="@T2@" ("搜索字符串"), replace string=w335) -> (result string=w330:string)  [unwired: 5 in, 3 out]
            n191 = local read "input_str_label"() -> (w329:string)
            n192 = local read "SDD11"() -> (w322:string)
            n193 = Search and Replace String(input string=w330, search string="@L@" ("搜索字符串"), replace string=w329) -> (result string=w325:string)  [unwired: 5 in, 3 out]
            n194 = local read "midVar_Content"() -> (w334:string)
            n195 = Search and Replace String(input string=w325, search string="@R@" ("搜索字符串"), replace string=w322) -> (result string=w324:string)  [unwired: 5 in, 3 out]
            n196 = Concatenate Strings(w334, w324) -> (w333:string)
            n197 = local write "midVar_Content"(w333) -> ()
          }
          frame "body_detail_SDD11" {
            n198 = local read "input_path_dataSource"() -> (w346:path)
            n199 = local read "input_str_label"() -> (w349:string)
            n200 = Build Path(base path=w346, name or relative path="TXT" ("名称或相对路径")) -> (appended path=w355:path)
            n201 = local read "single spec"() -> (w345:T1)
            n202 = local read "SDD11"() -> (w342:string)
            n203 = Build Path(base path=w355, name or relative path="SDD11.txt" ("名称或相对路径")) -> (appended path=w353:path)
            n204 = local read "midVar_Content"() -> (w348:string)
            n205 = call "get single spec.vi"("single item name"="SDD11", "single spec"=w345) -> ("single spec"=w343:dbl[])  [unwired: 9 in]
            n206 = call "xmlFull.vi"("TDD?"=FALSE, "second result"=w342, "file path (dialog if empty)"=w353, "limit type"=enum16{"上限", "下限"}."上限", "SN"=w349, "single spec"=w343, "数组"=string[] ["Port1-Port2: TD-RD", "Port1-Port2: RD-TD"]) -> ("OutPutXml"=w352:string)  [unwired: 3 in]
            n207 = Concatenate Strings(w348, w352) -> (w347:string)
            n208 = local write "midVar_Content"(w347) -> ()
          }
          frame "body_e_SDD11" {
            n209 = local read "midVar_Content"() -> (w361:string)
            n210 = Concatenate Strings(w361, "        </ItemTest>\n") -> (w360:string)
            n211 = local write "midVar_Content"(w360) -> ()
          }
          frame "body_s_SCD21-SDD21" {
            n212 = local read "midVar_time"() -> (w367:string[])
            n213 = local read "input_str_label"() -> (w369:string)
            n214 = Index Array(array=w367, index #1=2 ("索引"), index #2=3 ("索引")) -> (element #1=w378:string, element #2=w375:string)
            n215 = Search and Replace String(input string="        <ItemTest ID=\"6\" name=\"Jitter From (SCD21-SDD21)\" startDateTime=\"@T1@\" endDateTime=\"@T2@\">\n            <TestResult BoardFlag=\"1\" ID=\"1\" SerialNumber=\"@L@\" ValueFlag=\"0\">\n                <Outcome value=\"@R@\"/>\n                <Description>NoDesc</Description>\n            </TestResult>\n ", search string="@T1@" ("搜索字符串"), replace string=w378) -> (result string=w377:string)  [unwired: 5 in, 3 out]
            n216 = Search and Replace String(input string=w377, search string="@T2@" ("搜索字符串"), replace string=w375) -> (result string=w370:string)  [unwired: 5 in, 3 out]
            n217 = Search and Replace String(input string=w370, search string="@L@" ("搜索字符串"), replace string=w369) -> (result string=w365:string)  [unwired: 5 in, 3 out]
            n218 = local read "SCD21-SDD21"() -> (w362:string)
            n219 = Search and Replace String(input string=w365, search string="@R@" ("搜索字符串"), replace string=w362) -> (result string=w364:string)  [unwired: 5 in, 3 out]
            n220 = local read "midVar_Content"() -> (w374:string)
            n221 = Concatenate Strings(w374, w364) -> (w373:string)
            n222 = local write "midVar_Content"(w373) -> ()
          }
          frame "body_detail_SCD21-SDD21" {
            n223 = local read "input_path_dataSource"() -> (w390:path)
            n224 = local read "SCD21-SDD21"() -> (w385:string)
            n225 = local read "input_str_label"() -> (w389:string)
            n226 = Build Path(base path=w390, name or relative path="TXT" ("名称或相对路径")) -> (appended path=w394:path)
            n227 = local read "single spec"() -> (w384:T1)
            n228 = Build Path(base path=w394, name or relative path="SCD21-SDD21.txt" ("名称或相对路径")) -> (appended path=w392:path)
            n229 = call "get single spec.vi"("single item name"="SCD21-SDD21", "single spec"=w384) -> ("single spec"=w382:dbl[])  [unwired: 9 in]
            n230 = call "xmlFull.vi"("second result"=w385, "file path (dialog if empty)"=w392, "limit type"=enum16{"上限", "下限"}."上限", "SN"=w389, "single spec"=w382, "数组"=string[] ["Port1-Port2: TD-RD", "Port1-Port2: RD-TD"]) -> ("OutPutXml"=w391:string)  [unwired: 4 in]
            n231 = local read "midVar_Content"() -> (w387:string)
            n232 = Concatenate Strings(w387, w391) -> (w386:string)
            n233 = local write "midVar_Content"(w386) -> ()
          }
          frame "body_e_SCD21-SDD21" {
            n234 = local read "midVar_Content"() -> (w400:string)
            n235 = Concatenate Strings(w400, "        </ItemTest>\n") -> (w399:string)
            n236 = local write "midVar_Content"(w399) -> ()
          }
          frame "body_s_paddle card" {
            n237 = local read "midVar_time"() -> (w408:string[])
            n238 = Index Array(array=w408, index #1=2 ("索引"), index #2=3 ("索引")) -> (element #1=w416:string, element #2=w413:string)
            n239 = local read "input_str_label"() -> (w407:string)
            n240 = Search and Replace String(input string="        <ItemTest ID=\"7\" name=\"Differential Impedance Paddle card\" startDateTime=\"@T1@\" endDateTime=\"@T2@\">\n            <TestResult BoardFlag=\"1\" ID=\"1\" SerialNumber=\"@L@\" ValueFlag=\"0\">\n                <Outcome value=\"@R@\"/>\n                <Description>NoDesc</Description>\n            </TestResult>\n ", search string="@T1@" ("搜索字符串"), replace string=w416) -> (result string=w415:string)  [unwired: 5 in, 3 out]
            n241 = Search and Replace String(input string=w415, search string="@T2@" ("搜索字符串"), replace string=w413) -> (result string=w411:string)  [unwired: 5 in, 3 out]
            n242 = Search and Replace String(input string=w411, search string="@L@" ("搜索字符串"), replace string=w407) -> (result string=w404:string)  [unwired: 5 in, 3 out]
            n243 = local read "TDD"() -> (w401:string)
            n244 = local read "midVar_Content"() -> (w406:string)
            n245 = Search and Replace String(input string=w404, search string="@R@" ("搜索字符串"), replace string=w401) -> (result string=w403:string)  [unwired: 5 in, 3 out]
            n246 = Concatenate Strings(w406, w403) -> (w405:string)
            n247 = local write "midVar_Content"(w405) -> ()
          }
          frame "body_detail_paddle card" {
            n248 = local read "input_path_dataSource"() -> (w445:path)
            n249 = Build Path(base path=w445, name or relative path="TXT" ("名称或相对路径")) -> (appended path=w448:path)
            n250 = local read "input_str_label"() -> (w442:string)
            n251 = local read "TDD"() -> (w423:string)
            n252 = Build Path(base path=w445, name or relative path="TXT" ("名称或相对路径")) -> (appended path=w453:path)
            n253 = local read "show_impspec"() -> (w422:string[])
            n254 = Build Path(base path=w448, name or relative path="TDD22.txt" ("名称或相对路径")) -> (appended path=w446:path)
            n255 = Build Path(base path=w453, name or relative path="TDD11.txt" ("名称或相对路径")) -> (appended path=w451:path)
            n256 = Index Array(array=w422, index=0 ("索引")) -> (element=w420:string)
            n257 = local read "midVar_Content"() -> (w426:string)
            n258 = local read "terminal points"() -> (w439:dbl[])
            n259 = Index Array(array=w439, index #1=0 ("索引"), index #2=1 ("索引")) -> (element #1=w430:dbl, element #2=w436:dbl)
            n260 = Subtract(x=w436, y=w430) -> (x-y=w433:dbl)
            n261 = Multiply(x=w433, y=0.1) -> (x*y=w432:dbl)
            n262 = Multiply(x=w433, y=0.2) -> (x*y=w431:dbl)
            n263 = Add(x=w430, y=w432) -> (x+y=w429:dbl)
            n264 = Add(x=w430, y=w431) -> (x+y=w428:dbl)
            n265 = Build Array(w429, w428) -> (w427:dbl[])
            n266 = call "xmlFull.vi"("TDD?"=TRUE, "second result"=w423, "Points"=w427, "file path (dialog if empty)"=w446, "TDD spec"=w420, "SN"=w442, "数组"=string[] ["Paddle Card_TD:ZDD22", "Paddle Card_RD:ZDD22"]) -> ("OutPutXml"=w424:string)  [unwired: 3 in]
            n267 = call "xmlFull.vi"("TDD?"=TRUE, "second result"=w423, "Points"=w427, "file path (dialog if empty)"=w451, "TDD spec"=w420, "SN"=w442, "数组"=string[] ["Paddle Card_TD:ZDD11", "Paddle Card_RD:ZDD11"]) -> ("OutPutXml"=w450:string)  [unwired: 3 in]
            n268 = Concatenate Strings(w426, w450, w424) -> (w425:string)
            n269 = local write "midVar_Content"(w425) -> ()
          }
          frame "body_e_paddle card" {
            n270 = local read "midVar_Content"() -> (w458:string)
            n271 = Concatenate Strings(w458, "        </ItemTest>\n") -> (w457:string)
            n272 = local write "midVar_Content"(w457) -> ()
          }
          frame "body_s_ILD" {
            n273 = local read "midVar_time"() -> (w465:string[])
            n274 = Index Array(array=w465, index #1=3 ("索引"), index #2=4 ("索引")) -> (element #1=w476:string, element #2=w473:string)
            n275 = Search and Replace String(input string="        <ItemTest ID=\"8\" name=\"Insertion Loss Deviation\" startDateTime=\"@T1@\" endDateTime=\"@T2@\">\n            <TestResult BoardFlag=\"1\" ID=\"1\" SerialNumber=\"@L@\" ValueFlag=\"0\">\n                <Outcome value=\"@R@\"/>\n                <Description>NoDesc</Description>\n            </TestResult>\n ", search string="@T1@" ("搜索字符串"), replace string=w476) -> (result string=w475:string)  [unwired: 5 in, 3 out]
            n276 = Search and Replace String(input string=w475, search string="@T2@" ("搜索字符串"), replace string=w473) -> (result string=w468:string)  [unwired: 5 in, 3 out]
            n277 = local read "input_str_label"() -> (w467:string)
            n278 = local read "ILD"() -> (w460:string)
            n279 = Search and Replace String(input string=w468, search string="@L@" ("搜索字符串"), replace string=w467) -> (result string=w463:string)  [unwired: 5 in, 3 out]
            n280 = local read "midVar_Content"() -> (w472:string)
            n281 = Search and Replace String(input string=w463, search string="@R@" ("搜索字符串"), replace string=w460) -> (result string=w462:string)  [unwired: 5 in, 3 out]
            n282 = Concatenate Strings(w472, w462) -> (w471:string)
            n283 = local write "midVar_Content"(w471) -> ()
          }
          frame "body_detail_ILD" {
            n284 = local read "input_path_dataSource"() -> (w489:path)
            n285 = Build Path(base path=w489, name or relative path="TXT" ("名称或相对路径")) -> (appended path=w493:path)
            n286 = local read "input_str_label"() -> (w487:string)
            n287 = local read "ILD"() -> (w484:string)
            n288 = local read "single spec"() -> (w483:T1)
            n289 = local read "midVar_Content"() -> (w485:string)
            n290 = Build Path(base path=w493, name or relative path="ILD.txt" ("名称或相对路径")) -> (appended path=w491:path)
            n291 = call "get single spec.vi"("single item name"="ILD", "single spec"=w483) -> ("single spec"=w481:dbl[])  [unwired: 9 in]
            n292 = call "xmlFull.vi"("second result"=w484, "file path (dialog if empty)"=w491, "limit type"=enum16{"上限", "下限"}."上限", "SN"=w487, "single spec"=w481, "数组"=string[] ["Port1-Port2: TD-RD", "Port1-Port2: RD-TD"], "ABS?"=TRUE) -> ("OutPutXml"=w490:string)  [unwired: 3 in]
            n293 = Concatenate Strings(w485, w490) -> (w486:string)
            n294 = local write "midVar_Content"(w486) -> ()
          }
          frame "body_e_ILD" {
            n295 = local read "midVar_Content"() -> (w499:string)
            n296 = Concatenate Strings(w499, "        </ItemTest>\n") -> (w498:string)
            n297 = local write "midVar_Content"(w498) -> ()
          }
          frame "tail" {
            # "</ResultSet>\n    <TestProgram Productline=\"XT-113\" Product=\"SFP+\">\n        <c:Definition name=\"HPTS\" version=\"6.0\">\n            <c:Description>NoDesc</c:Description> \n        </c:Definition>\n    </TestProgram>\n    <!--  ATE--> \n    <TestStation AteName=\"TDR\" AteVersion=\"1.001\" /> \n    <!--  SerialNumber--> \n    <UUT UutType=\"hardware\">\n        <SerialNumber>@L@</SerialNumber> \n        <ItemName>SFP+</ItemName>\n        <ItemCode>@C@</ItemCode> \n    </UUT>\n    <WorkOrder>\n        <WorkItem name=\"a\">\n            <c:Datum xsi:type=\"c:string\">\n                <c:Value>SPZS06311C1</c:Value> \n            </c:Datum>\n        </WorkItem>\n    </WorkOrder>\n</TestResults"
            n298 = Concatenate Strings("\"" ("字符串"), "FileVer", "\"" ("字符串")) -> (w504:string)
            n299 = local read "input_str_product"() -> (w526:string)
            n300 = Search and Replace String(input string="    </ResultSet>\n    <TestProgram Productline=\"XT-113\" Product=\"SFP+\">\n        <c:Definition name=\"VNA\" version=@Ver@>\n            <c:Description>@Path@</c:Description> \n        </c:Definition>\n    </TestProgram>\n    <!--  ATE--> \n    <TestStation AteName=@PCName@ AteVersion=\"1.001\" /> \n    <!--  SerialNumber--> \n    <UUT UutType=\"hardware\">\n        <SerialNumber>@L@</SerialNumber> \n        <ItemName>SFP+</ItemName>\n        <ItemCode>@C@</ItemCode> \n    </UUT>\n    <WorkOrder>\n        <WorkItem name=\"a\">\n            <c:Datum xsi:type=\"c:string\">\n                <c:Value>SPZS06311C1</c:Value> \n            </c:Datum>\n        </WorkItem>\n    </WorkOrder>\n</TestResults>", search string="@Ver@" ("搜索字符串"), replace string=w504) -> (result string=w513:string)  [unwired: 5 in, 3 out]
            n301 = call "PCsName.vi"() -> ("Computer Name"=w503:string)
            n302 = Search and Replace String(input string=w513, search string="@Path@" ("搜索字符串"), replace string="FilePath") -> (result string=w511:string)  [unwired: 5 in, 3 out]
            n303 = local read "input_str_label"() -> (w523:string)
            n304 = Concatenate Strings("\"" ("字符串"), w503, "\"" ("字符串")) -> (w500:string)
            n305 = Search and Replace String(input string=w511, search string="@PCName@" ("搜索字符串"), replace string=w500) -> (result string=w509:string)  [unwired: 5 in, 3 out]
            n306 = Search and Replace String(input string=w509, search string="@P@" ("搜索字符串"), replace string=w526) -> (result string=w525:string)  [unwired: 5 in, 3 out]
            n307 = Search and Replace String(input string=w525, search string="@L@" ("搜索字符串"), replace string=w523) -> (result string=w518:string)  [unwired: 5 in, 3 out]
            n308 = local read "input_str_CustomerPN"() -> (w516:string)
            n309 = local read "midVar_Content"() -> (w522:string)
            n310 = Search and Replace String(input string=w518, search string="@C@" ("搜索字符串"), replace string=w516) -> (result string=w519:string)  [unwired: 5 in, 3 out]
            n311 = Concatenate Strings(w522, w519) -> (w521:string)
            n312 = local write "midVar_Content"(w521) -> ()
          }
          frame "end" {
            n313 = local read "midVar_Content"() -> (w529:string)
            n314 = Open/Create/Replace File(file path (use dialog)="路径", operation (0:open)=T2."open or create" ("操作(0:open)")) -> (refnum out=w533:refnum<file>)  [unwired: 4 in, 2 out]
            n315 = Text to UTF-8(11:w529) -> (3:w528:string)  [unwired: 1 in, 1 out]
            n316 = Write to Text File(file (use dialog)=w533, text=w528) -> (refnum out=w532:refnum<file>)  [unwired: 2 in, 2 out]
            n317 = Close File(refnum=w532) -> ()  [unwired: 1 in, 2 out]
          }
        }
        n318 = local write "midVar_state"(w68) -> ()
      }
    }
  }
